vi "FG GPS Trail Bearing.vi"(1 "FG Action (Read)":T1, 2 "GPS Trail Bearing in":dbl) -> (0 "GPS Trail Bearing out":dbl)   [LabVIEW 2009]
uses:
  Actions for FG's.ctl
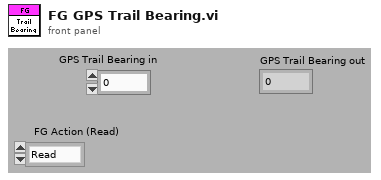
[diagram p1: front panel]
types:
  T1 = typedef "Actions for FG's.ctl" = enum16{"Read", "Write"}
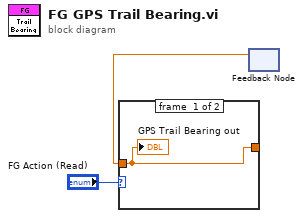
[diagram p0: block diagram]
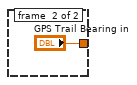
[diagram p2: hidden frame]
diagram:
  n1 = feedback #1() -> (w1:dbl)  [unwired: 1 in]
  n2 = case shown="\"Write\"" "FG Action (Read)" {
    tunnel: [w4 "GPS Trail Bearing in"] -> w2
    tunnel: w1 -> [w4 _]
    frame #0 {
      "GPS Trail Bearing out" <- w4
    }
    frame #1 {
    }
  }
